vi "Groups.vi"(8 "error in (no error)":errorcluster, 11 "Task in":refnum<class "Task.lvclass">) -> (0 "error out":errorcluster, 2 "Groups":refnum<class "Group.lvclass">[](array[class]), 3 "Task out":refnum<class "Task.lvclass">)   [LabVIEW 2020, in "VolatusConfig.lvlib" / "Task.lvclass"]
uses:
  Task.lvclass
  Task.lvclass/Task.ctl
  lv-cdm/CDM-Config/Config Element/Config Element.lvclass
  lv-cdm/CDM-Config/Config Manager/Config Manager.lvclass
  VolatusConfig.lvlib
  Meta Type.ctl
  Group/Group.lvclass
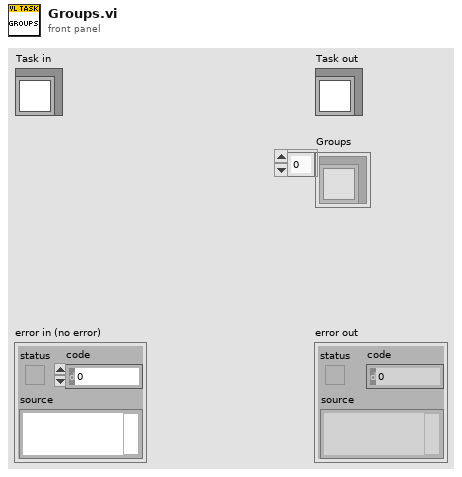
[diagram p1: front panel]
types:
  T1 = typedef "VolatusConfig.lvlib/Meta Type.ctl" = enum16{"VL_System", "VL_Cluster", "VL_Node", "VL_Task", "VL_Group", "VL_Channel"}
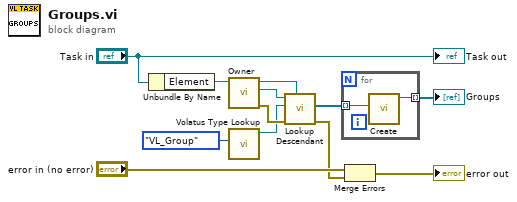
[diagram p0: block diagram]
diagram:
  n1 = Unbundle By Name("Task in") -> ("Element"=w10:refnum<class "Config Element.lvclass">)
  n2 = call "Owner.vi"("Config Element in"=w10) -> ("error out"=w7:errorcluster, "Owner"=w9:refnum<class "Config Manager.lvclass">, "Config Element out"=w8:refnum<class "Config Element.lvclass">)  [unwired: 8 in]
  n3 = call "Volatus Type Lookup.vi"("Meta Type"=Meta_Type."VL_Group") -> ("Config Lookup out"=w6:refnum<class "Config Lookup.lvclass">)  [unwired: 9 in, 1 out]
  n4 = call "Lookup Descendant.vi"("Start (Root)"=w8, "error in (no error)"=w7, "Lookup"=w6, "Config Manager in"=w9) -> ("error out"=w1:errorcluster, "Descendants"=w4:refnum<class "Config Element.lvclass">[])  [unwired: 5 in, 1 out]
  n5 = for {
    tunnel: w4 -> [w14] mode=indexing
    tunnel: [w13] -> w3 mode=indexing
    n6 = call "Create.vi"("Element"=w14) -> ("Group out"=w13:refnum<class "Group.lvclass">)  [unwired: 9 in, 1 out]
  }
  "Groups" <- w3
  n7 = Merge Errors("error in (no error)", w1) -> (→"error out":errorcluster)
  "Task out" <- "Task in"
